vi "Add Port RTM.vi"(8 "error in":errorcluster, 11 "Node Ptr":u64 format="%.0x") -> (0 "error out":errorcluster)   [LabVIEW 2020, in "Communication Bus Template System Explorer.lvlib"]
doc: "This VI runs when the Add Port run-time menu is chosen. It allows the user to create a port with an associated database."
uses:
  Communication Bus Template System Explorer.lvlib
  <vilib>/NI VeriStand/Custom Device Tools/Custom Device Utility Library/Search Direction.ctl
  <vilib>/NI VeriStand/Custom Device API/Custom Device Item Ref.ctl
  Shared/Constants.vi
  <vilib>/NI VeriStand/Custom Device Tools/Custom Device Utility Library/NI VeriStand - Search for Item by GUID.vi
  <vilib>/NI VeriStand/Custom Device API/Set Item Property (String).vi
  <vilib>/NI VeriStand/Custom Device API/Set Item Property (Path).vi
  <vilib>/NI VeriStand/Custom Device API/Set Item Property (U32).vi
  <vilib>/NI VeriStand/Custom Device API/Get Item Property (Path).vi
  Shared/Communication Bus Template Shared.lvlib
  <vilib>/NI VeriStand/Custom Device Tools/Custom Device Utility Library/Custom Device Utility Library.lvlib
  <vilib>/NI VeriStand/Custom Device API/Custom Device API.lvlib
panel:
  in  "Baud Rate":u32
  in  "Database":string(combo)
  in  "Port Name":string
  in  "Help":bool
  in  "Cancel":bool
  in  "OK":bool
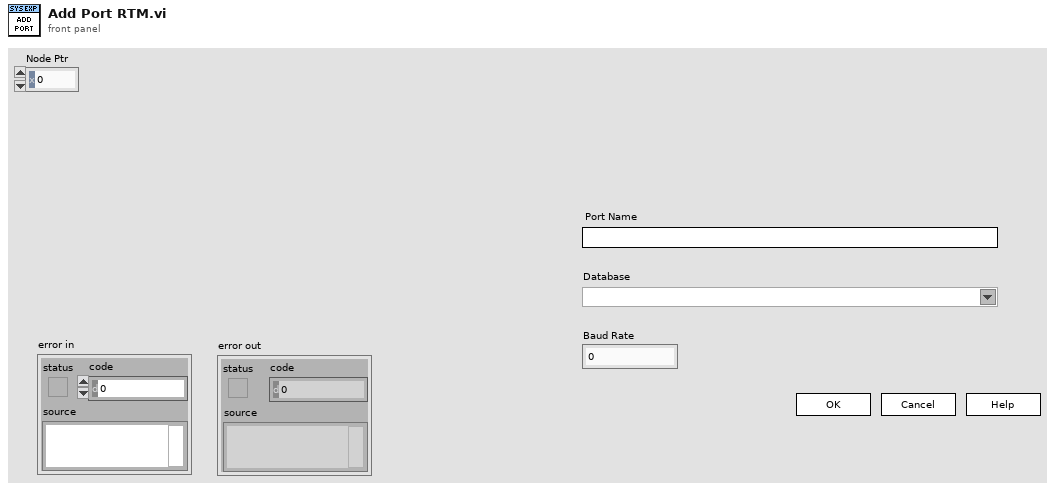
[diagram p1: front panel]
types:
  T1 = typedef "Custom Device Utility Library.lvlib/Search Direction.ctl" = enum16{"Down", "Up"}
  T2 = typedef "Custom Device API.lvlib/Custom Device Item Ref.ctl" = u64
  T3 = cluster{"Baud Rate":u32, "Port Name":string, "Database Name":string, "Database Path":path, "Databases ref":T2, "Node Ptr":u64}
  T4 = typedef "Custom Device API.lvlib/Custom Device Item Info.ctl" = cluster{"Name":string, "Is Channel":bool, "GUID":string, "Is Waveform":bool}
  T5 = typedef "Communication Bus Template System Explorer.lvlib/Database.ctl" = cluster{"Baud Rate":u64, "Frames":cluster{"Name":string, "ID":i32}[]}
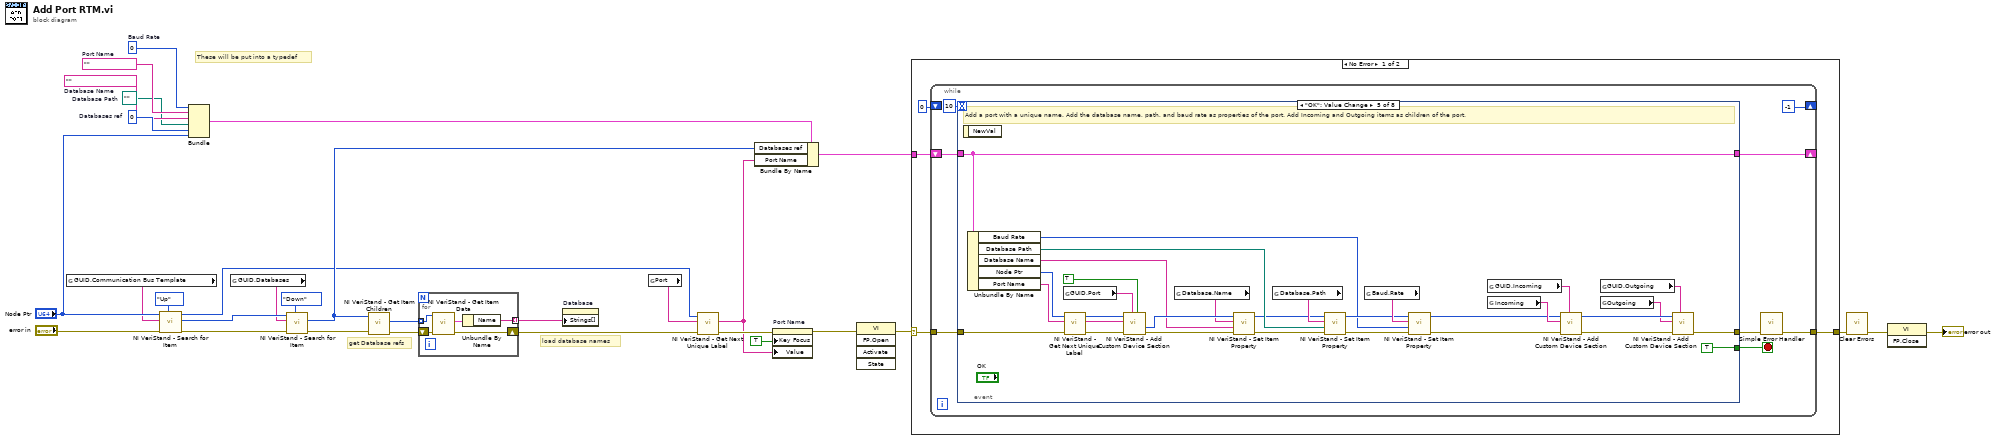
[diagram p0: block diagram]
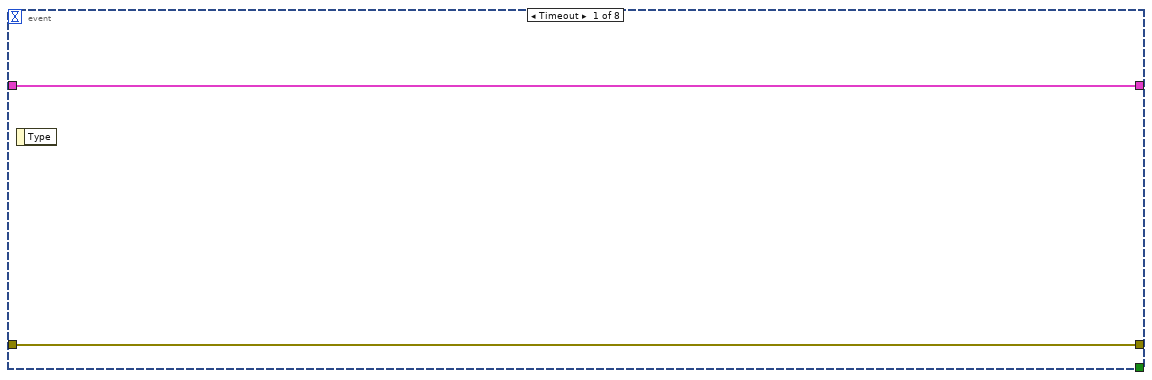
[diagram p2: hidden frame]
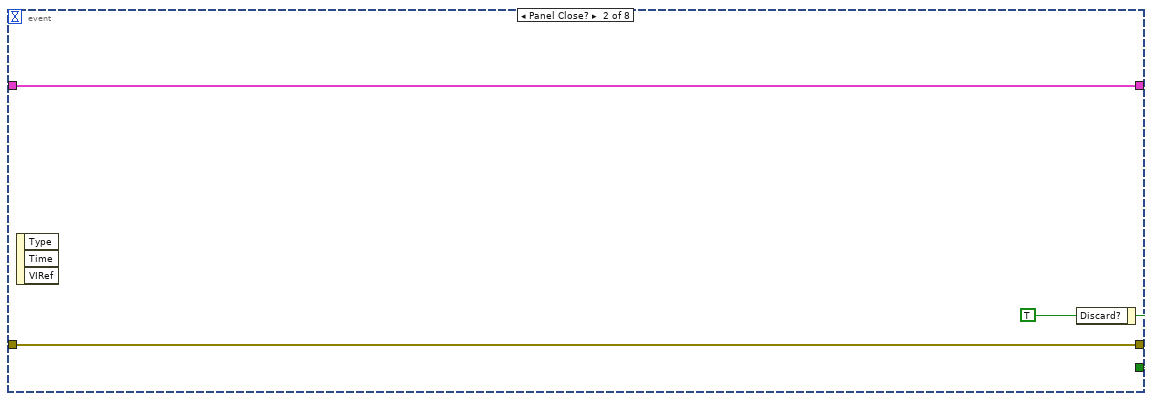
[diagram p3: hidden frame]
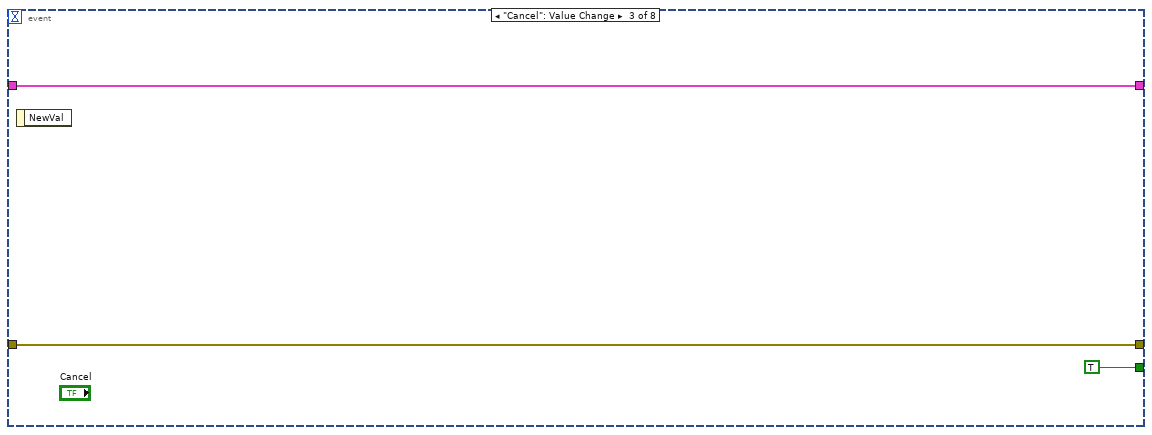
[diagram p4: hidden frame]
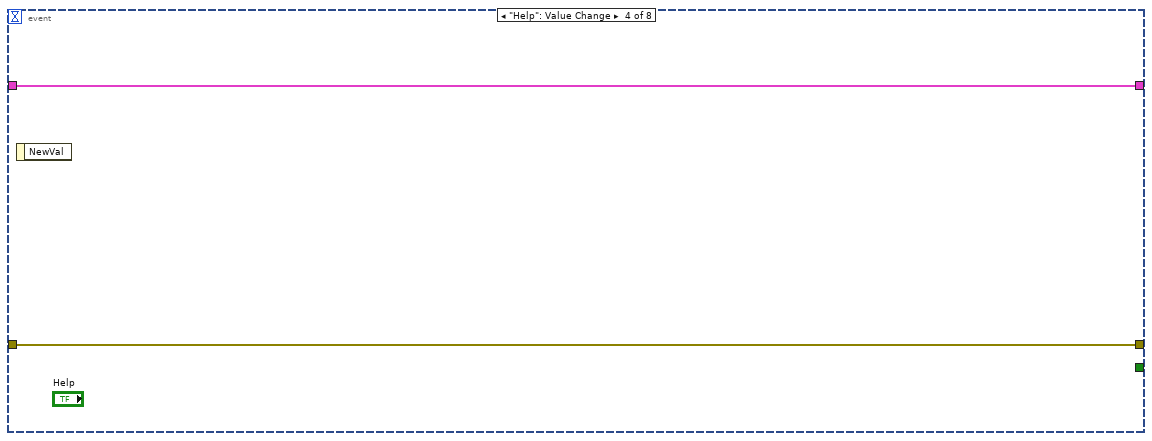
[diagram p5: hidden frame]
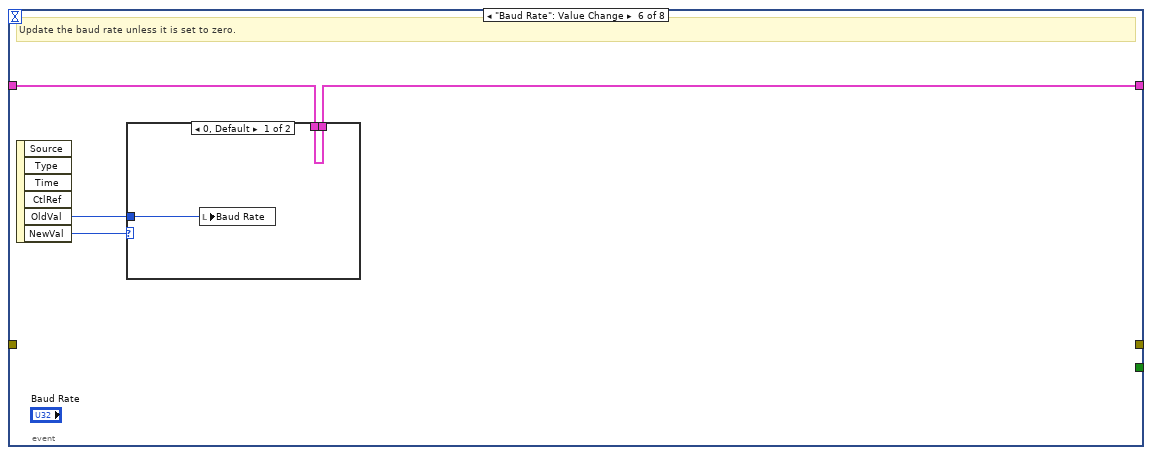
[diagram p6: hidden frame]
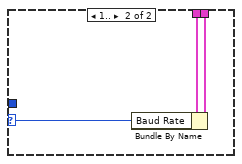
[diagram p7: hidden frame]
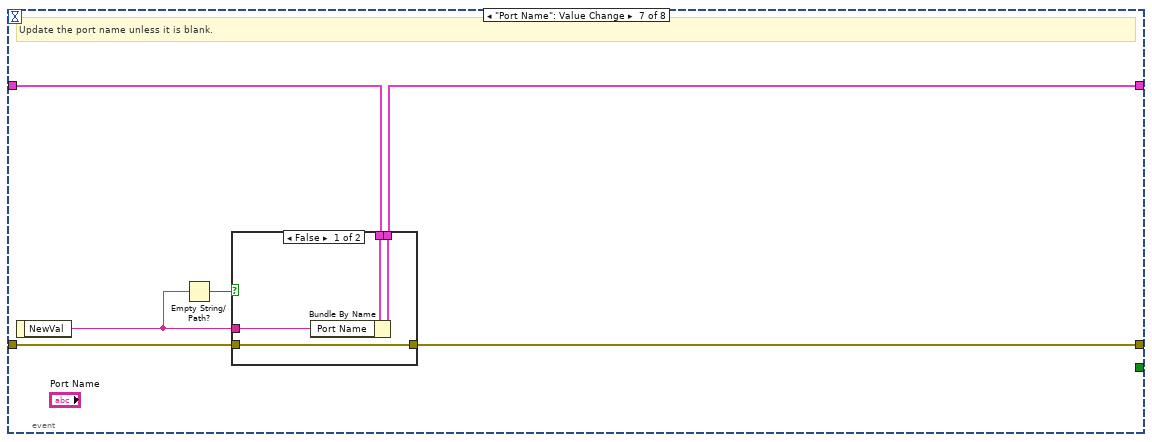
[diagram p8: hidden frame]
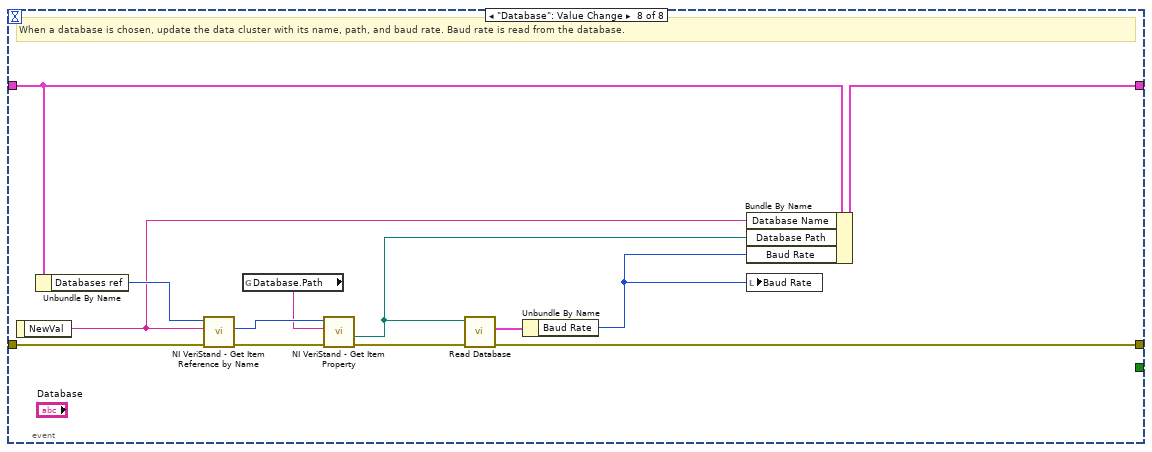
[diagram p10: hidden frame]
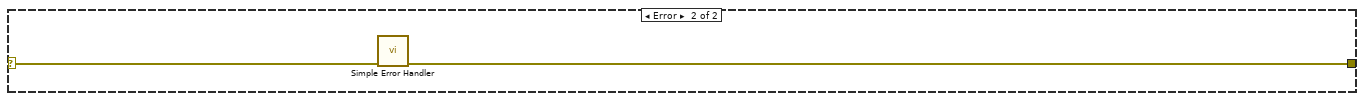
[diagram p11: hidden frame]
diagram:
  w4 = u32 0  # Baud Rate
  w6 = path ""  # Database Path
  w8 = ""  # Database Name
  w14 = T2 0  # Databases ref
  w7 = ""  # Port Name
  # "These will be put into a typedef"
  # "load database names"
  # "get Database refs"
  n1 = global read "Constants.vi" "GUID.Communication Bus Template"() -> (w3:string)
  n2 = call-poly <vilib>:"NI VeriStand - Search for Item.vi"("Direction (Down)"=Search_Direction."Up", "error in"="error in", "Item GUID"=w3, "Section Ref in"="Node Ptr") -> ("error out"=w17:errorcluster, "Item Ref"=w16:T2, "Section Ref out"=w11:T2)  [unwired: 4 in, 1 out]
  n3 = Bundle("Baud Rate"=w4, "Port Name"=w7, "Database Name"=w8, "Database Path"=w6, "Databases ref"=w14, "Node Ptr"="Node Ptr") -> (w22:T3)  [unwired: 1 in]
  n4 = global read "Constants.vi" "GUID.Databases"() -> (w5:string)
  n5 = call-poly <vilib>:"NI VeriStand - Search for Item.vi"("Direction (Down)"=Search_Direction."Down", "error in"=w17, "Item GUID"=w5, "Section Ref in"=w16) -> ("error out"=w18:errorcluster, "Item Ref"=w13:T2)  [unwired: 4 in, 2 out]
  n6 = call <vilib>:"NI VeriStand - Get Item Children.vi"("error in (no error)"=w18, "Item Ref in"=w13) -> ("error out"=w20:errorcluster, "Child Refs"=w19:T2[])  [unwired: 6 in, 2 out]
  n7 = for {
    tunnel: w19 -> [w35] mode=indexing
    shift-right: [w33] -> w15
    shift-left: w20 -> [w34]
    tunnel: [w32] -> w21 mode=indexing
    n8 = call <vilib>:"NI VeriStand - Get Item Data.vi"("error in (no error)"=w34, "Item Ref in"=w35) -> ("error out"=w33:errorcluster, "Item Info"=w36:T4)  [unwired: 6 in, 2 out]
    n9 = Unbundle By Name(w36) -> ("Name"=w32:string)
  }
  n10 = property on="Database" class="CmbBox"("Strings[]"=w21) -> ()  [unwired: 2 in, 2 out]
  n11 = global read "Constants.vi" "Port"() -> (w23:string)
  n12 = call <vilib>:"NI VeriStand - Get Next Unique Label.vi"("error in (no error)"=w15, "Label"=w23, "Parent Ref in"=w11) -> ("error out"=w24:errorcluster, "Label out"=w12:string)  [unwired: 5 in, 2 out]
  n13 = Bundle By Name(cluster=w22, "Databases ref"=w13, "Port Name"=w12) -> (w29:T3)
  n14 = property on="Port Name" class="Str"(error in=w24, "Key Focus"=TRUE, "Value"=w12) -> (error out=w28:errorcluster)  [unwired: 1 in, 1 out]
  n15 = invoke class="VI" method="FP.Open"(error in=w28) -> (error out=w27:errorcluster)  [unwired: 4 in, 4 out]
  n16 = case shown="No Error" w27 {
    selector: w27 -> [w40 w125]
    tunnel: [w39 w124] -> w30
    tunnel: w29 -> [w37 _]
    frame No Error {
      n17 = while {
        tunnel: w40 -> [w48]
        tunnel: [w46] -> w39
        shift-right: [-1] -> _
        shift-left: 0 -> [_]
        shift-right: [w42] -> _
        shift-left: w37 -> [w43]
        stop <- w45 stop-if-true
        n18 = event shown="[4] \"OK\": Value Change" {
          selector: _ -> [_ _ _ _ _ _ _ _]
          dyn-events: _ -> [_ _ _ _ _ _ _ _]
          timeout: 10 -> [_ _ _ _ _ _ _ _]
          tunnel: [w50 w53 w55 w58 w73 _ w103 w114] -> w47
          tunnel: w48 -> [w50 w53 w55 w58 w85 _ w104 w122]
          tunnel: [_ w52 TRUE ("Discard?") _ TRUE ("Discard?") _ _ _] -> w45
          tunnel: w43 -> [w49 w51 w54 w57 w82 w91 w100 w121]
          tunnel: [w49 w51 w54 w57 w82 w92 w99 w123] -> w42
          event Timeout {
            n19 = event-data() -> ()  [unwired: 1 in, 1 out]
          }
          event Panel Close? {
            w52 = TRUE ("Discard?")
            n20 = event-data() -> ()  [unwired: 1 in, 3 out]
            n21 = event-data("Discard?"=w52) -> ()  [unwired: 1 in, 1 out]
          }
          event "Cancel": Value Change {
            n22 = event-data() -> ()  [unwired: 1 in, 1 out]
          }
          event "Help": Value Change {
            n23 = event-data() -> ()  [unwired: 1 in, 1 out]
          }
          event "OK": Value Change {
            # "Add a port with a unique name. Add the database name, path, and baud rate as properties of the port. Add Incoming and Outgoing items as children of the port."
            n24 = event-data() -> ()  [unwired: 1 in, 1 out]
            n25 = Unbundle By Name(w82) -> ("Baud Rate"=w59:u32, "Database Path"=w67:path, "Database Name"=w70:string, "Node Ptr"=w81:u64, "Port Name"=w80:string)
            n26 = global read "Constants.vi" "GUID.Port"() -> (w87:string)
            n27 = call <vilib>:"NI VeriStand - Get Next Unique Label.vi"("error in (no error)"=w85, "Label"=w80, "Parent Ref in"=w81) -> ("error out"=w86:errorcluster, "Label out"=w83:string, "Parent Ref dup"=w84:T2)  [unwired: 5 in, 1 out]
            n28 = call <vilib>:"NI VeriStand - Add Custom Device Section.vi"("Highlight? (F)"=TRUE, "GUID (Default Section)"=w87, "error in (no error)"=w86, "Section Name"=w83, "Parent Ref in"=w84) -> ("error out"=w71:errorcluster, "Section Ptr"=w72:T2)  [unwired: 3 in, 2 out]
            n29 = global read "Constants.vi" "Database.Name"() -> (w69:string)
            n30 = call-poly <vilib>:"NI VeriStand - Set Item Property.vi"("error in (no error)"=w71, "Value"=w70, "Property Name"=w69, "Item Ref in"=w72) -> ("error out"=w66:errorcluster, "Item Ref out"=w65:T2)  [unwired: 5 in, 1 out]
            n31 = global read "Constants.vi" "Database.Path"() -> (w68:string)
            n32 = call-poly <vilib>:"NI VeriStand - Set Item Property.vi"("error in (no error)"=w66, "Value"=w67, "Property Name"=w68, "Item Ref in"=w65) -> ("error out"=w60:errorcluster, "Item Ref out"=w63:T2)  [unwired: 5 in, 1 out]
            n33 = global read "Constants.vi" "Baud.Rate"() -> (w64:string)
            n34 = call-poly <vilib>:"NI VeriStand - Set Item Property.vi"("error in (no error)"=w60, "Value"=w59, "Property Name"=w64, "Item Ref in"=w63) -> ("error out"=w61:errorcluster, "Item Ref out"=w62:T2)  [unwired: 5 in, 1 out]
            n35 = global read "Constants.vi" "GUID.Incoming"() -> (w74:string)
            n36 = global read "Constants.vi" "Incoming"() -> (w75:string)
            n37 = call <vilib>:"NI VeriStand - Add Custom Device Section.vi"("GUID (Default Section)"=w74, "error in (no error)"=w61, "Section Name"=w75, "Parent Ref in"=w62) -> ("error out"=w79:errorcluster, "Parent Ref out"=w78:T2)  [unwired: 4 in, 2 out]
            n38 = global read "Constants.vi" "GUID.Outgoing"() -> (w77:string)
            n39 = global read "Constants.vi" "Outgoing"() -> (w76:string)
            n40 = call <vilib>:"NI VeriStand - Add Custom Device Section.vi"("GUID (Default Section)"=w77, "error in (no error)"=w79, "Section Name"=w76, "Parent Ref in"=w78) -> ("error out"=w73:errorcluster)  [unwired: 4 in, 3 out]
          }
          event "Baud Rate": Value Change {
            # "Update the baud rate unless it is set to zero."
            n41 = event-data() -> ("OldVal"=w90:u32, "NewVal"=w93:u32)  [unwired: 1 in, 4 out]
            n42 = case shown="0, Default" w93 {
              selector: w93 -> [_ w96]
              tunnel: w91 -> [w95 w98]
              tunnel: [w95 w97] -> w92
              tunnel: w90 -> [w94 _]
              frame 0, Default {
                n43 = local write "Baud Rate"(w94) -> ()
              }
              frame 1.. {
                n44 = Bundle By Name(cluster=w98, "Baud Rate"=w96) -> (w97:T3)
              }
            }
          }
          event "Port Name": Value Change {
            # "Update the port name unless it is blank."
            n45 = event-data() -> ("NewVal"=w101:string)  [unwired: 1 in]
            n46 = Empty String/Path?(string/path=w101) -> (empty?=w102:bool)
            n47 = case shown="False" w102 {
              tunnel: w104 -> [w108 w110]
              tunnel: w101 -> [w106 _]
              tunnel: [w108 w110] -> w103
              tunnel: w100 -> [w107 w109]
              tunnel: [w105 w109] -> w99
              frame False {
                n48 = Bundle By Name(cluster=w107, "Port Name"=w106) -> (w105:T3)
              }
              frame True {
              }
            }
          }
          event "Database": Value Change {
            # "When a database is chosen, update the data cluster with its name, path, and baud rate. Baud rate is read from the database."
            n49 = event-data() -> ("NewVal"=w116:string)  [unwired: 1 in]
            n50 = Unbundle By Name(w121) -> ("Databases ref"=w120:T2)
            n51 = call <vilib>:"NI VeriStand - Get Item Reference by Name.vi"("error in (no error)"=w122, "Item Name"=w116, "Parent Ref in"=w120) -> ("error out"=w119:errorcluster, "Item Ref"=w118:T2)  [unwired: 5 in, 2 out]
            n52 = global read "Constants.vi" "Database.Path"() -> (w117:string)
            n53 = call-poly <vilib>:"NI VeriStand - Get Item Property.vi"("error in (no error)"=w119, "Property Name"=w117, "Item Ref in"=w118) -> ("error out"=w115:errorcluster, "Value"=w113:path)  [unwired: 5 in, 2 out]
            n54 = call "Read Database.vi"("error in"=w115, "Path"=w113) -> ("error out"=w114:errorcluster, "Database"=w112:T5)  [unwired: 8 in]
            n55 = Unbundle By Name(w112) -> ("Baud Rate"=w111:u64)
            n56 = Bundle By Name(cluster=w121, "Database Name"=w116, "Database Path"=w113, "Baud Rate"=w111) -> (w123:T3)
            n57 = local write "Baud Rate"(w111) -> ()
          }
        }
        n58 = call <vilib>:"Simple Error Handler.vi"("error in (no error)"=w47) -> ("error out"=w46:errorcluster)  [unwired: 4 in, 4 out]
      }
    }
    frame Error {
      n59 = call <vilib>:"Simple Error Handler.vi"("error in (no error)"=w125) -> ("error out"=w124:errorcluster)  [unwired: 4 in, 4 out]
    }
  }
  n60 = call <vilib>:"Clear Errors.vi"("error in (no error)"=w30) -> ("error out"=w26:errorcluster)  [unwired: 5 in, 1 out]
  n61 = invoke class="VI" method="FP.Close"(error in=w26) -> (error out=→"error out":errorcluster)  [unwired: 2 in, 2 out]
